vi "core_vi_name_regex.vi"() -> (0 "regex":string="([ \\w-()\\.]+\\.lvlib)?:?([ \\w-()\\.]+)(\\.vi|\\.ctl):?([Ii]nstance:\\d+)?")   [LabVIEW 2015]
doc: "Four capturing groups:\n1. Library name with extension (zero or one time)\n2. vi/ctrl name\n3. vi/ctrl extension\n4. Instance number (zero or one time)\nhttps://regex101.com/"
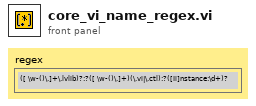
[diagram p1: front panel]
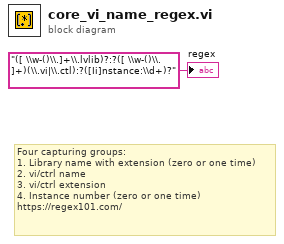
[diagram p0: block diagram]
diagram:
  # "Four capturing groups:\n1. Library name with extension (zero or one time)\n2. vi/ctrl name\n3. vi/ctrl extension\n4. Instance number (zero or one time)\nhttps://regex101.com/"
  "regex" <- "([ \\w-()\\.]+\\.lvlib)?:?([ \\w-()\\.]+)(\\.vi|\\.ctl):?([Ii]nstance:\\d+)?" ("regex")
